vi "FPGA manager.vi"(5 "force":bool, 7 "action":T2, 8 "error in":errorcluster, 9 "bitfile to cache":refnum<k20>, 10 "Bitfile path":path, 11 "RIO resource":T1 caption="RIO Device") -> (0 "error out":errorcluster, 1 "found?":bool, 3 "bitfile":refnum<k20>)   [LabVIEW 2013, in "FPGA manager.lvlib"]
uses:
  FPGA manager.lvlib
  methods.ctl
  <vilib>/userdefined/High Color/nirio_resource_hc.ctl
  <vilib>/Utility/error.llb/Error Cluster From Error Code.vi
  <vilib>/FPGAPlugInAG/Dynamic/niLvFpga_Close_Dynamic.vi
  <vilib>/ErrorRing/Error Ring.xnode
  <vilib>/rvi/interface/nirviCloseFPGA/nirviCloseFPGA.xnode
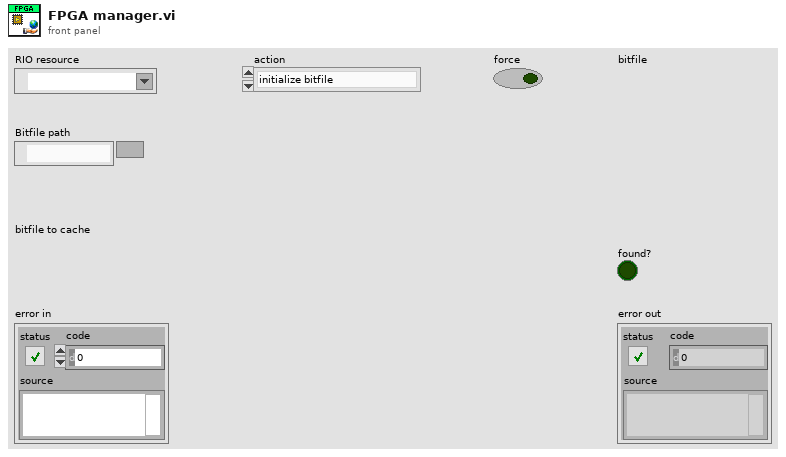
[diagram p1: front panel]
types:
  T1 = typedef "nirio_resource_hc.ctl" = tag
  T2 = typedef "FPGA manager.lvlib/methods.ctl" = enum16{"initialize bitfile", "cache bitfile", "locate bitfile", "close bitfile"}
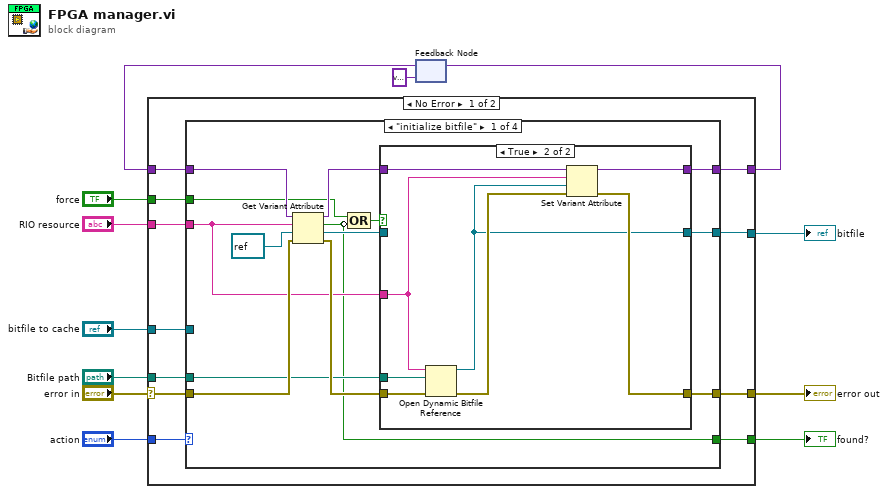
[diagram p0: block diagram]
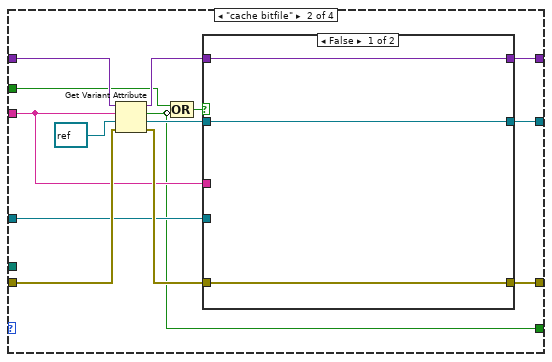
[diagram p3: hidden frame]
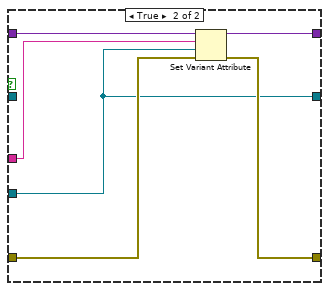
[diagram p4: hidden frame]
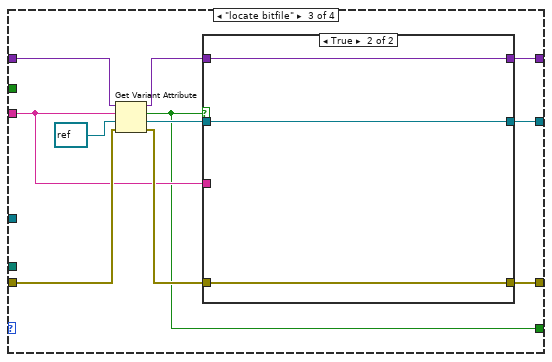
[diagram p5: hidden frame]
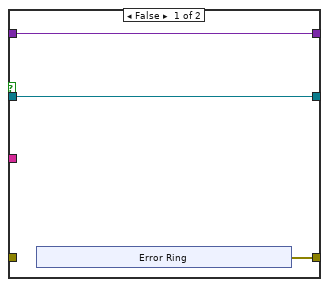
[diagram p6: hidden frame]
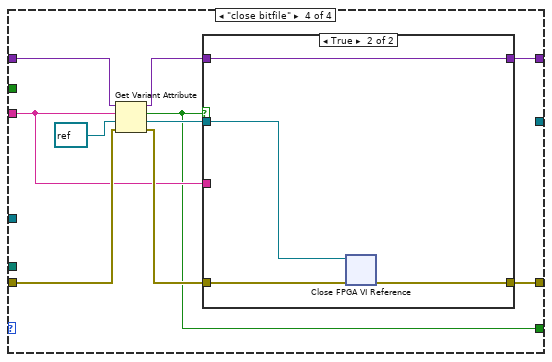
[diagram p7: hidden frame]
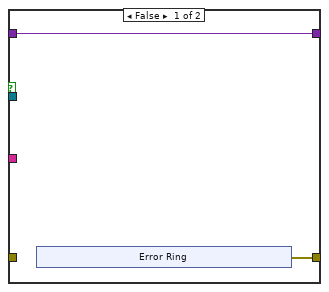
[diagram p8: hidden frame]
diagram:
  n1 = feedback #1(variant) -> (w6:variant)
  n2 = case shown="No Error" "error in" {
    selector: "error in" -> [w22 w114]
    tunnel: [w18 w114] -> w11
    tunnel: "action" -> [w23 _]
    tunnel: "RIO resource" -> [w21 _]
    tunnel: [w20 _] -> w9
    tunnel: "force" -> [w19 _]
    tunnel: [w17 w113] -> w7
    tunnel: w6 -> [w16 w113]
    tunnel: "Bitfile path" -> [w15 _]
    tunnel: "bitfile to cache" -> [w14 _]
    tunnel: [w13 _] -> w2
    frame No Error {
      n3 = case shown="\"initialize bitfile\"" w23 {
        tunnel: w22 -> [w34 w59 w79 w100]
        tunnel: w21 -> [w25 w51 w73 w94]
        tunnel: [w36 w61 w81 _] -> w20
        tunnel: w19 -> [w27 w53 _ _]
        tunnel: [w31 w56 w76 w97] -> w18
        tunnel: [w30 w55 w75 w96] -> w17
        tunnel: w16 -> [w29 w54 w74 w95]
        tunnel: w15 -> [w28 _ _ _]
        tunnel: w14 -> [_ w50 _ _]
        tunnel: [w24 w49 w72 w93] -> w13
        frame "initialize bitfile" {
          n4 = Get Variant Attribute(Variant=w29, name=w25, default value (empty Variant)=refnum<k20> refnum ("Bitfile reference out"), error in=w34) -> (duplicate Variant=w32:variant, found=w24:bool, value=w35:refnum<k20>, error out=w33:errorcluster)
          n5 = Compound Arithmetic op=OR(w27, invert w24) -> (w26:bool)
          n6 = case shown="True" w26 {
            tunnel: [w40 w41] -> w36
            tunnel: w35 -> [w40 _]
            tunnel: w33 -> [w39 w48]
            tunnel: w32 -> [w38 w43]
            tunnel: [w39 w45] -> w31
            tunnel: [w38 w46] -> w30
            tunnel: w28 -> [_ w47]
            tunnel: w25 -> [_ w42]
            frame False {
            }
            frame True {
              n7 = Open Dynamic Bitfile Reference(0:w42, 1:w47, 3:w48) -> (5:w41:refnum<k20>, 8:w44:errorcluster)  [unwired: 2 in]
              n8 = Set Variant Attribute(Variant=w43, name=w42, value=w41, error in=w44) -> (Variant out=w46:variant, error out=w45:errorcluster)  [unwired: 1 out]
            }
          }
        }
        frame "cache bitfile" {
          n9 = Get Variant Attribute(Variant=w54, name=w51, default value (empty Variant)=refnum<k20> refnum ("Bitfile reference out"), error in=w59) -> (duplicate Variant=w57:variant, found=w49:bool, value=w60:refnum<k20>, error out=w58:errorcluster)
          n10 = Compound Arithmetic op=OR(w53, invert w49) -> (w52:bool)
          n11 = case shown="False" w52 {
            tunnel: [w65 w66] -> w61
            tunnel: w60 -> [w65 _]
            tunnel: w58 -> [w64 w71]
            tunnel: w57 -> [w63 w68]
            tunnel: [w64 w69] -> w56
            tunnel: [w63 w70] -> w55
            tunnel: w51 -> [_ w67]
            tunnel: w50 -> [_ w66]
            frame False {
            }
            frame True {
              n12 = Set Variant Attribute(Variant=w68, name=w67, value=w66, error in=w71) -> (Variant out=w70:variant, error out=w69:errorcluster)  [unwired: 1 out]
            }
          }
        }
        frame "locate bitfile" {
          n13 = Get Variant Attribute(Variant=w74, name=w73, default value (empty Variant)=refnum<k20> refnum ("Bitfile reference out"), error in=w79) -> (duplicate Variant=w77:variant, found=w72:bool, value=w80:refnum<k20>, error out=w78:errorcluster)
          n14 = case shown="True" w72 {
            tunnel: [w84 w92] -> w81
            tunnel: w80 -> [w84 w92]
            tunnel: w78 -> [_ w91]
            tunnel: w77 -> [w85 w90]
            tunnel: [w83 w91] -> w76
            tunnel: [w85 w90] -> w75
            tunnel: w73 -> [_ _]
            frame False {
              n15 = xnode "Error Ring"() -> ("error out"=w83:errorcluster)
            }
            frame True {
            }
          }
        }
        frame "close bitfile" {
          n16 = Get Variant Attribute(Variant=w95, name=w94, default value (empty Variant)=refnum<k20> refnum ("Bitfile reference out"), error in=w100) -> (duplicate Variant=w98:variant, found=w93:bool, value=w101:refnum<k20>, error out=w99:errorcluster)
          n17 = case shown="True" w93 {
            tunnel: w101 -> [_ w109]
            tunnel: w99 -> [_ w111]
            tunnel: w98 -> [w104 w112]
            tunnel: [w103 w110] -> w97
            tunnel: [w104 w112] -> w96
            tunnel: w94 -> [_ _]
            frame False {
              n18 = xnode "Error Ring"() -> ("error out"=w103:errorcluster)
            }
            frame True {
              n19 = xnode "Close FPGA VI Reference"("FPGA VI Reference In"=w109, "error in"=w111) -> ("error out"=w110:errorcluster)
            }
          }
        }
      }
    }
    frame Error {
    }
  }
  "error out" <- w11
  "bitfile" <- w9
  "found?" <- w2
  n20 = feedback-in #1(w7) -> ()
